vi "Destroy Logger(by Ref).vi"(8 "error in (no error)":errorcluster) -> (0 "error out":errorcluster)   [LabVIEW 2017, in "Error Log.lvlib" / "Logger.lvclass"]
doc: "Closes all handlers and removes them from the referenced Logger and destrois the reference to the Logger."
uses:
  Logger.lvclass
  Logger.lvclass/Logger.ctl
  Get Handlers.vi
  Handler/Handler.lvclass
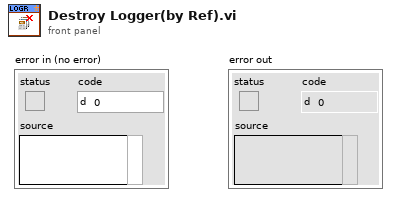
[diagram p1: front panel]
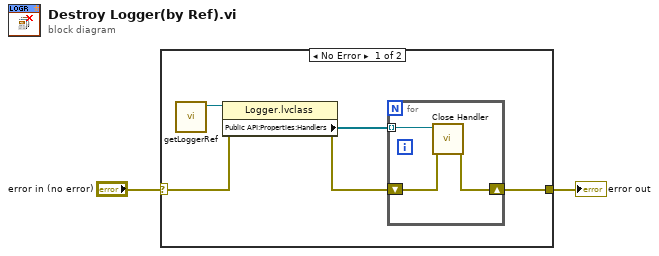
[diagram p0: block diagram]
diagram:
  n1 = case shown="No Error" "error in (no error)" {
    selector: "error in (no error)" -> [w4 w11]
    tunnel: [w7 w11] -> w1
    frame No Error {
      n2 = call "getLoggerRef.vi"() -> ("Logger Ref"=w3:refnum<data-value>)  [unwired: 10 in, 1 out]
      n3 = property class="Logger.lvclass"(reference=w3, error in=w4) -> (error out=w5:errorcluster, "Public API:Properties:Handlers"=w6:refnum<class "Handler.lvclass">[])  [unwired: 1 out]
      n4 = for {
        tunnel: w6 -> [w10] mode=indexing
        shift-right: [w8] -> w7
        shift-left: w5 -> [w9]
        n5 = call "Close Handler.vi"("error in (no error)"=w9, "Handler in"=w10) -> ("error out"=w8:errorcluster)  [unwired: 8 in, 1 out]
      }
    }
    frame Error {
    }
  }
  "error out" <- w1
